vi "CreateCasarti.vi"(11 "Input Array":csg[][][](array[numeric])) -> (3 "output array":csg[][](array[numeric]))   [LabVIEW 2022 SP3]
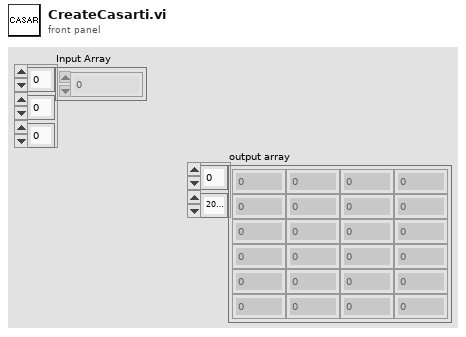
[diagram p1: front panel]
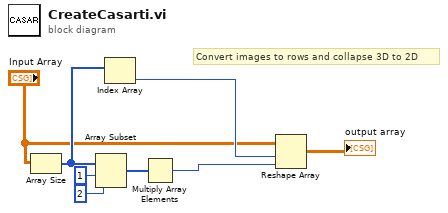
[diagram p0: block diagram]
diagram:
  # "Convert images to rows and collapse 3D to 2D"
  n1 = Array Size(array="Input Array") -> (size(s)=w4:i32[])
  n2 = Array Subset(array=w4, index=1, length=2) -> (w8:i32[])
  n3 = Index Array(array=w4) -> (element=w3:i32)  [unwired: 1 in]
  n4 = Multiply Array Elements(1:w8) -> (0:w5:i32)
  n5 = Reshape Array("Input Array", w3, w5) -> (→"output array":csg[][])
